vi "Relay control.vi"() -> ()   [LabVIEW 2009]
doc: "Sets the AFG3252 (function generator) to sweep through three specified frequency ranges, at a given overall repetition rate. (Used for resonating the nuclei.) Takes advantage of the FM sweep mode of the function generator. Outputs on channel 1 and uses channel 2 to trigger the relays."
uses:
  <vilib>/Platform/TimedLoop/XDataNode/wakeup.ctl
  <vilib>/Platform/TimedLoop/XDataNode/XDNodeRunTimeDep.lvlib
  <vilib>/Platform/TimedLoop/XDataNode/nitl_modes.ctl
  <vilib>/Platform/TimedLoop/XDataNode/timing_clust.ctl
  <vilib>/Platform/TimedLoop/XDataNode/XDataNode.xnode
  <vilib>/DAQmx/write.llb/DAQmx Write (Digital 1D Bool 1Chan 1Samp).vi
  <vilib>/Platform/TimedLoop/XDataNode/loadlvalarms.vi
  <vilib>/DAQmx/create/timing.llb/DAQmx Create Timing Source (Digital Edge using Counter).vi
  <vilib>/DAQmx/create/channels.llb/DAQmx Create Channel (DO-Digital Output).vi
  FG FM sweep center span control.ctl
  FG FM sweep start stop control.ctl
panel:
  in  "set":bool
  in  "start/stop":T1 {"stop" min=0.0 step=10000.0 format="%.2g"; "start" min=0.0 step=10000.0 format="%.2g"}
  out "Global Start Time":u64=130100113623490
  in  "center/span":T2 {"span" min=0.0 step=10000.0 format="%.2g"; "center" min=0.0 step=10000.0 format="%.2g"}
  in  "exit":bool
  in  "Overall rep rate":dbl[unit]=50.0 min=0.0 step=0.01 format="%.2g"
  # "For instructions on how to configure the cables correctly for the function generator, see the block diagram."
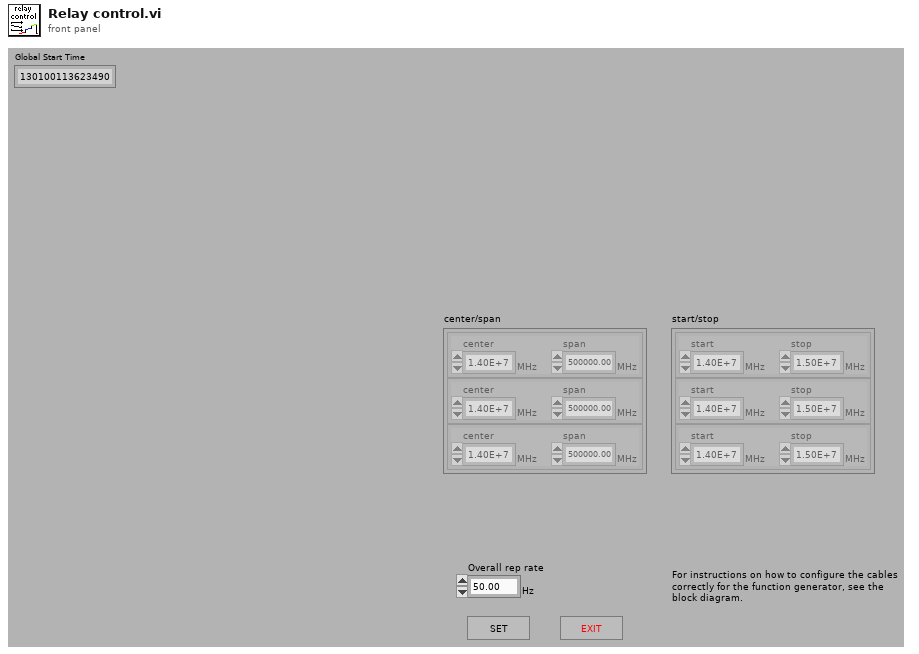
[diagram p1: front panel]
types:
  T1 = typedef "FG FM sweep start stop control.ctl" = cluster{"start":dbl[unit], "stop":dbl[unit]}[]
  T2 = typedef "FG FM sweep center span control.ctl" = cluster{"center":dbl[unit], "span":dbl[unit]}[]
  T3 = cluster{cluster{dbl, dbl}, cluster{dbl, dbl}, cluster{dbl, dbl}}
  T4 = typedef "XDNodeRunTimeDep.lvlib/timing_clust.ctl" = cluster{"Expected End [f-1]":u64, "Actual End [f-1]":u64, "Finished Late? [f-1]":bool, "Expected End [i-1]":u64, "Actual End [i-1]":u64, "Finished Late? [i-1]":bool, "Expected Start [i]":u64, "Actual Start [i]":u64, "Expected Start [f]":u64, "Actual Start [f]":u64, "Source Name":string, "Structure Name":string, "Period":i64, "Deadline":i64, "Offset":i64, "Start":i64, "Priority":i32, "Timeout":i32, "Mode":T5, "Wakeup Reason":T6, "Error":errorcluster, "Source Type":string, "Secondary Source Type":string, "Global End Time":u64, "Global Start Time":u64, "Frame Duration":u64, "Iteration Duration":u64, "Assigned CPU":i32, "I/O Scan Engine Mode":u32}
  T5 = typedef "XDNodeRunTimeDep.lvlib/nitl_modes.ctl" = enum32{"No Change", "Process missed periods, maintain original phase", "Discard missed periods, maintain original phase", "Process missed periods, ignore original phase", "Discard missed periods, ignore original phase"}
  T6 = typedef "XDNodeRunTimeDep.lvlib/wakeup.ctl" = enum32{"Normal", "Aborted", "Asynchronous wakeup", "Timing source error", "Timed loop error", "Timeout"}
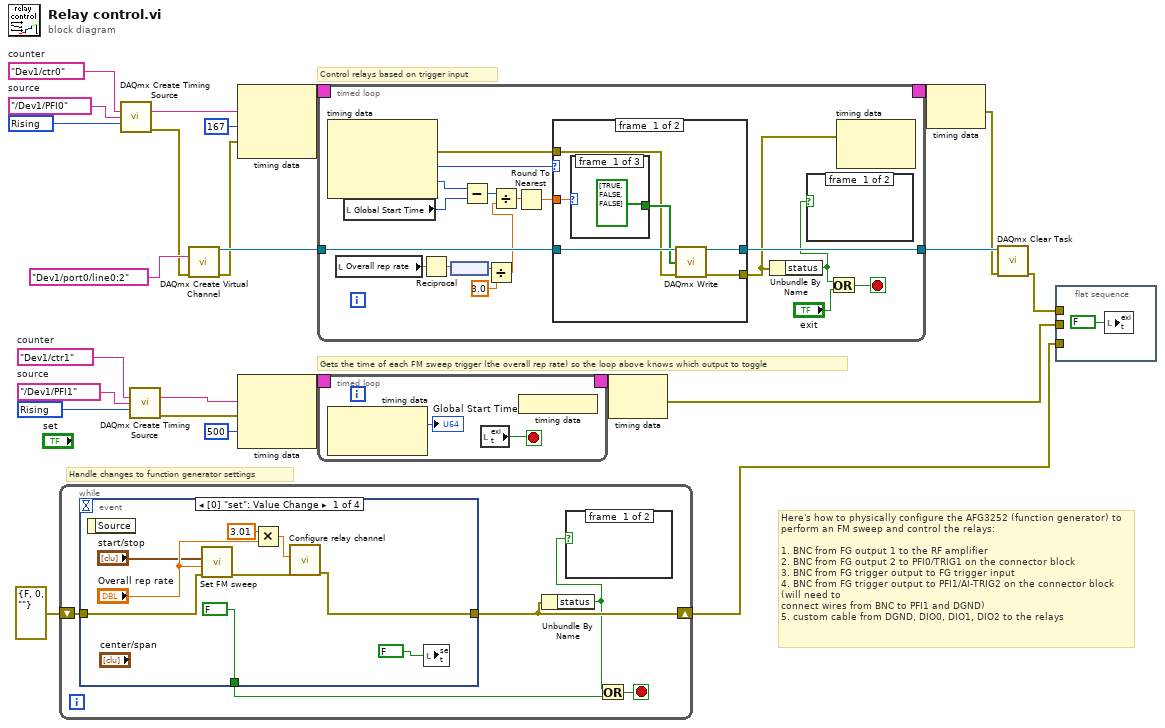
[diagram p0: block diagram]
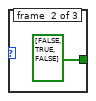
[diagram p2: hidden frame]
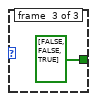
[diagram p3: hidden frame]
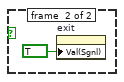
[diagram p5: hidden frame]
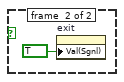
[diagram p6: hidden frame]
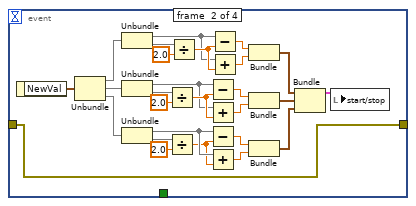
[diagram p7: hidden frame]
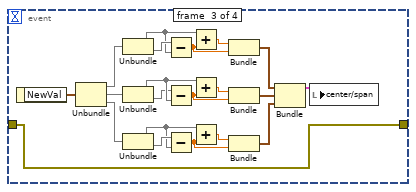
[diagram p8: hidden frame]
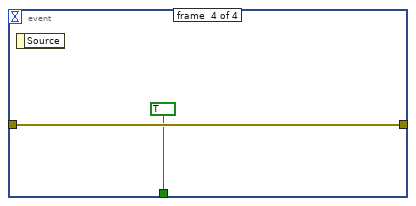
[diagram p9: hidden frame]
diagram:
  w15 = 10280 items=["Rising"=10280, "Falling"=10171] ("edge")
  w13 = tag "/Dev1/PFI1"  # source
  w14 = tag "Dev1/ctr1"  # counter
  w18 = 10280 items=["Rising"=10280, "Falling"=10171] ("edge")
  w20 = tag "/Dev1/PFI0"  # source
  w19 = tag "Dev1/ctr0"  # counter
  # "Here's how to physically configure the AFG3252 (function generator) to perform an FM sweep and control the relays:\n\n1. BNC from FG output 1 to the RF amplifier\n2. BNC from FG output 2 to PFI0/TRIG1 on the connector block\n3. BNC from FG trigger output to FG trigger input\n4. BNC from FG trigger output to PFI1/AI-TRIG2 on the connector block (will need to \nconnect wires from BNC to PFI1 and DGND)\n5. custom cable from DGND, DIO0, DIO1, DIO2 to the relays"
  # "Gets the time of each FM sweep trigger (the overall rep rate) so the loop above knows which output to toggle"
  # "Control relays based on trigger input"
  # "Handle changes to function generator settings"
  n1 = while {
    shift-right: [w29] -> w6
    shift-left: errorcluster {"status"=FALSE, "code"=0, "source"=""} ("error in (no error)") -> [w30]
    stop <- w26 stop-if-true
    n2 = event shown="[0] \"set\": Value Change" {
      selector: _ -> [_ _ _ _]
      dyn-events: _ -> [_ _ _ _]
      timeout: _ -> [_ _ _ _]
      tunnel: [FALSE _ _ TRUE] -> w27
      tunnel: w30 -> [w39 w41 w68 w90]
      tunnel: [w34 w41 w68 w90] -> w29
      event #0 {
        n3 = event-data() -> ()  [unwired: 2 out]
        n4 = call "Set FM sweep.vi"("error in (no error)"=w39, "# frequencies"="Overall rep rate", "Start/stop frequencies"="start/stop") -> ("error out"=w35:errorcluster)  [unwired: 2 in, 6 out]
        n5 = Multiply(x=3.01, y="Overall rep rate") -> (x*y=w36:dbl[unit])
        n6 = call "Configure relay channel.vi"("error in (no error)"=w35, "relay frequency"=w36) -> ("error out"=w34:errorcluster)  [unwired: 1 in, 8 out]
        n7 = local write "set"(FALSE) -> ()
      }
      event #1 {
        n8 = event-data() -> ("NewVal"=w42:T2)  [unwired: 1 out]
        n9 = Unbundle(w42) -> (w67, w66, w65)
        n10 = Unbundle(w67) -> (w54, w53)
        n11 = Unbundle(w66) -> (w58, w57)
        n12 = Unbundle(w65) -> (w62, w63)
        n13 = Divide(x=w57, y=2.0) -> (x/y=w60:dbl)
        n14 = Divide(x=w63, y=2.0) -> (x/y=w61:dbl)
        n15 = Divide(x=w53, y=2.0) -> (x/y=w55:dbl)
        n16 = Subtract(x=w58, y=w60) -> (x-y=w50:dbl)
        n17 = Add(x=w58, y=w60) -> (x+y=w49:dbl)
        n18 = Subtract(x=w62, y=w61) -> (x-y=w48:dbl)
        n19 = Add(x=w62, y=w61) -> (x+y=w47:dbl)
        n20 = Subtract(x=w54, y=w55) -> (x-y=w52:dbl)
        n21 = Add(x=w54, y=w55) -> (x+y=w51:dbl)
        n22 = Bundle(w52, w51) -> (w46:cluster{dbl, dbl})  [unwired: 1 out]
        n23 = Bundle(w50, w49) -> (w45:cluster{dbl, dbl})  [unwired: 1 out]
        n24 = Bundle(w48, w47) -> (w44:cluster{dbl, dbl})  [unwired: 1 out]
        n25 = Bundle(w46, w45, w44) -> (w43:T3)  [unwired: 1 out]
        n26 = local write "start/stop"(w43) -> ()
      }
      event #2 {
        n27 = event-data() -> ("NewVal"=w69:T1)  [unwired: 1 out]
        n28 = Unbundle(w69) -> (w88, w79, w76)
        n29 = Unbundle(w88) -> (w82, w83)
        n30 = Unbundle(w79) -> (w81, w80)
        n31 = Unbundle(w76) -> (w77, w78)
        n32 = Subtract(x=w83, y=w82) -> (x-y=w74:dbl)
        n33 = Subtract(x=w80, y=w81) -> (x-y=w72:dbl)
        n34 = Subtract(x=w78, y=w77) -> (x-y=w70:dbl)
        n35 = Add(x=w82, y=w74) -> (x+y=w75:dbl)
        n36 = Add(x=w81, y=w72) -> (x+y=w73:dbl)
        n37 = Add(x=w77, y=w70) -> (x+y=w71:dbl)
        n38 = Bundle(w75, w74) -> (w87:cluster{dbl, dbl})  [unwired: 1 out]
        n39 = Bundle(w73, w72) -> (w86:cluster{dbl, dbl})  [unwired: 1 out]
        n40 = Bundle(w71, w70) -> (w85:cluster{dbl, dbl})  [unwired: 1 out]
        n41 = Bundle(w87, w86, w85) -> (w84:T3)  [unwired: 1 out]
        n42 = local write "center/span"(w84) -> ()
      }
      event #3 {
        n43 = event-data() -> ()  [unwired: 2 out]
      }
    }
    n44 = Unbundle By Name(w29) -> ("status"=w28:bool)
    n45 = case shown="True" w28 {
      frame #0 {
      }
      frame #1 {
        n46 = property on="exit" class="Bool (strict)"("Val(Sgnl)"=TRUE ("Value (Signaling)")) -> ()  [unwired: 2 in, 2 out]
      }
    }
    n47 = Or(x=w28, y=w27) -> (x .or. y?=w26:bool)
  }
  n48 = call-poly <vilib>:"DAQmx Create Timing Source.vi"("counter"=w19, "source"=w20, "edge"=w18) -> ("timing source out"=w17:string, "error out"=w9:errorcluster)  [unwired: 3 in, 8 out]
  n49 = call-poly <vilib>:"DAQmx Create Timing Source.vi"("counter"=w14, "source"=w13, "edge"=w15) -> ("timing source out"=w16:string, "error out"=w7:errorcluster)  [unwired: 3 in, 8 out]
  n50 = call-poly <vilib>:"DAQmx Create Virtual Channel.vi"("lines"=tag "Dev1/port0/line0:2", "error in"=w9) -> ("task out"=w10:refnum<k21>, "error out"=w8:errorcluster)  [unwired: 3 in, 9 out]
  n51 = node-c288(w17, 167 ("Timeout"), w8) -> (w24:T4)
  n52 = node-c288(w16, w7, 500 ("Timeout")) -> (w22:T4)
  n53 = timed-loop "Timed Loop" {
    timing-out: [_] -> w23
    timing: w24 -> [_]
    tunnel: w10 -> [w103]
    tunnel: [w102] -> w5
    stop <- w92 stop-if-true
    n54 = node-c288() -> (w101:errorcluster, w91:T6, w108:i64)  [unwired: 2 out]
    n55 = local read "Overall rep rate"() -> (w100:dbl[unit])
    n56 = local read "Global Start Time"() -> (w107:u64)
    n57 = Reciprocal(x=w100) -> (1/x=w98:dbl[unit])
    n58 = node(w98) -> (w99:dbl)
    n59 = Subtract(x=w108, y=w107) -> (x-y=w106:u64)
    n60 = Divide(x=w99, y=3.0) -> (x/y=w96:dbl)
    n61 = Divide(x=w106, y=w96) -> (x/y=w105:dbl)
    n62 = Round To Nearest(number=w105) -> (nearest integer value=w104:dbl)
    n63 = case shown="\"Normal\"" w91 {
      tunnel: w104 -> [w114 _]
      tunnel: w103 -> [w113 w119]
      tunnel: [w111 w119] -> w102
      tunnel: w101 -> [w110 w118]
      tunnel: [w109 w118] -> w95
      frame #0 {
        n64 = case shown="0, 3, Default" w114 {
          tunnel: [bool[] [TRUE, FALSE, FALSE] bool[] [FALSE, TRUE, FALSE] bool[] [FALSE, FALSE, TRUE]] -> w112
          frame #0 {
          }
          frame #1 {
          }
          frame #2 {
          }
        }
        n65 = call-poly <vilib>:"DAQmx Write.vi"("task/channels in"=w113, "data"=w112, "error in"=w110) -> ("task out"=w111:refnum<k21>, "error out"=w109:errorcluster)  [unwired: 1 in, 10 out]
      }
      frame #1 {
      }
    }
    n66 = Unbundle By Name(w95) -> ("status"=w94:bool)
    n67 = case shown="True" w94 {
      frame #0 {
      }
      frame #1 {
        n68 = property on="exit" class="Bool (strict)"("Val(Sgnl)"=TRUE ("Value (Signaling)")) -> ()  [unwired: 2 in, 2 out]
      }
    }
    n69 = Or(x=w94, y="exit") -> (x .or. y?=w92:bool)
    n70 = node-c288(w95) -> ()  [unwired: 2 out]
  }
  n71 = timed-loop "Timed Loop" {
    timing-out: [_] -> w21
    timing: w22 -> [_]
    stop <- w128 stop-if-true
    n72 = node-c288() -> (→"Global Start Time":i64)  [unwired: 2 out]
    n73 = local read "exit"() -> (w128:bool)
    n74 = node-c288() -> ()  [unwired: 1 out]
  }
  n75 = node-c288(w21) -> (w12:errorcluster)
  n76 = node-c288(w23) -> (w4:errorcluster)
  n77 = call <vilib>:"DAQmx Clear Task.vi"("task in"=w5, "error in"=w4) -> ("error out"=w3:errorcluster)  [unwired: 13 out]
  n78 = flat-sequence {
    tunnel: w12 -> [_]
    tunnel: w6 -> [_]
    tunnel: w3 -> [_]
    frame #0 {
      n79 = local write "exit"(FALSE ("exit")) -> ()
    }
  }
